vi "CacheConfigFile-SMTPAuthentication.vi"() -> (2 "Authentication Credentials":T1)   [LabVIEW 2020]
uses:
  SMTPCredentials.ctl
  Anemometry Sub Vis/Globals/Constants_global.vi
  <vilib>/Utility/config.llb/Read Key (String).vi
  <vilib>/Utility/config.llb/Write Key (String).vi
  <vilib>/Utility/config.llb/NI_LVConfig.lvlib
panel:
  out "file path":path
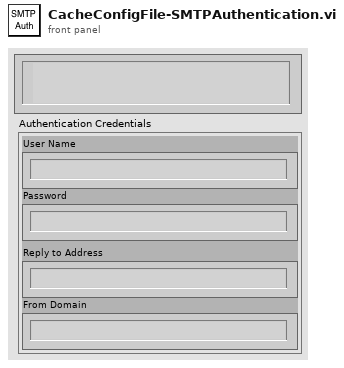
[diagram p1: front panel]
types:
  T1 = typedef "SMTPCredentials.ctl" = cluster{"User Name":string, "Password":string, "Reply to Address":string, "From Domain":string}
  T2 = typedef "NI_LVConfig.lvlib/Config Data RefNum.ctl" = refnum<k1>
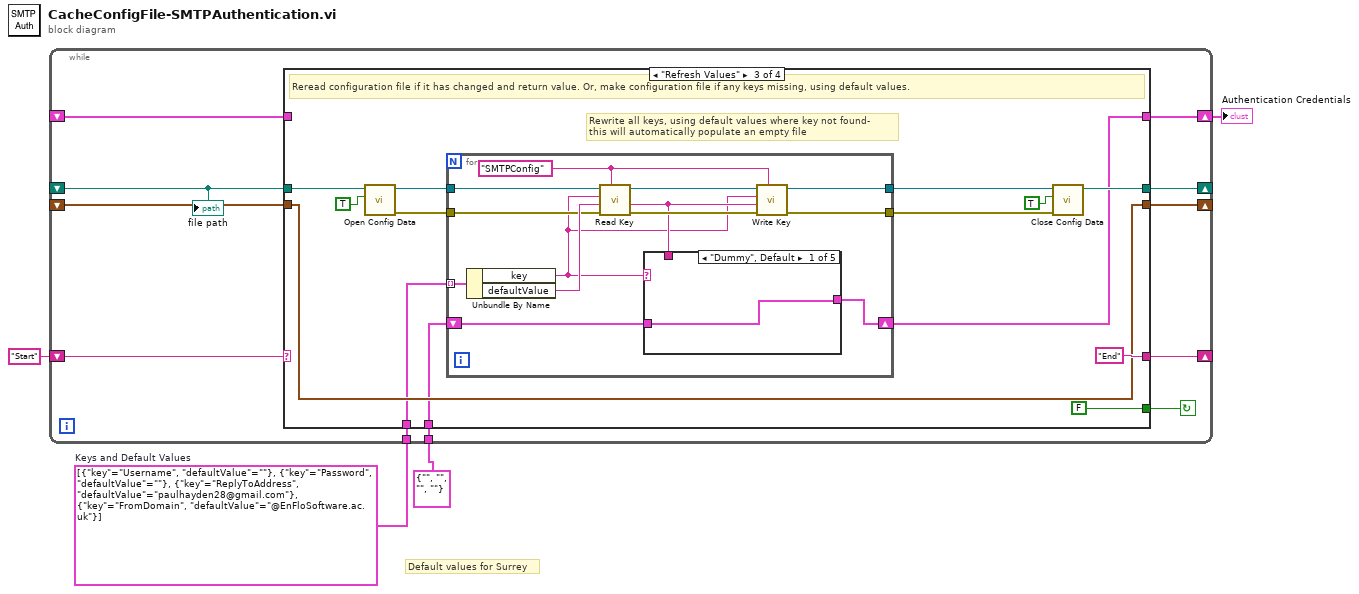
[diagram p0: block diagram]
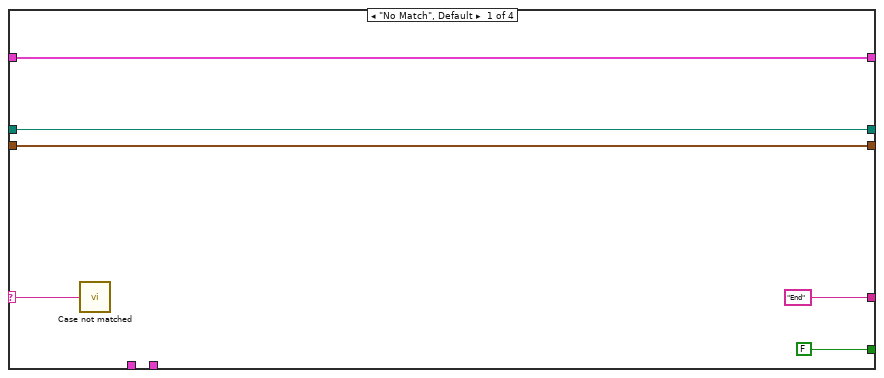
[diagram p2: hidden frame]
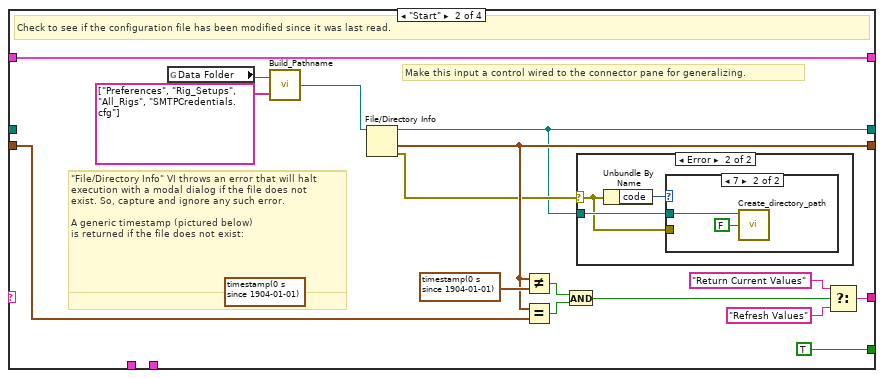
[diagram p3: hidden frame]
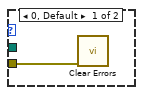
[diagram p5: hidden frame]
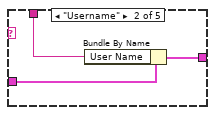
[diagram p6: hidden frame]
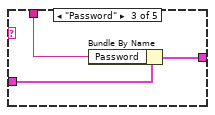
[diagram p7: hidden frame]
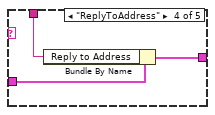
[diagram p8: hidden frame]
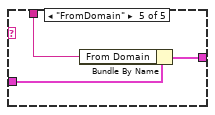
[diagram p9: hidden frame]
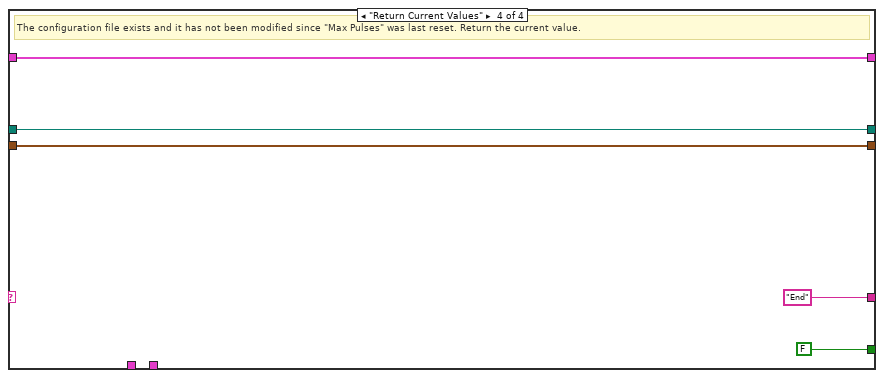
[diagram p10: hidden frame]
diagram:
  w2 = cluster{"key":string, "defaultValue":string}[] [{"key"="Username", "defaultValue"=""}, {"key"="Password", "defaultValue"=""}, {"key"="ReplyToAddress", "defaultValue"="paulhayden28@gmail.com"}, {"key"="FromDomain", "defaultValue"="@EnFloSoftware.ac.uk"}]  # Keys and Default Values
  # "Default values for Surrey"
  n1 = while {
    shift-left: _ -> [w9]
    shift-right: [w11] -> _
    shift-left: _ -> [w10]
    shift-right: [w12] -> w3
    shift-left: "Start" -> [w13]
    shift-right: [w14] -> _
    shift-right: [w8] -> _
    shift-left: _ -> [w7]
    tunnel: w2 -> [w6]
    tunnel: T1 {"User Name"="", "Password"="", "Reply to Address"="", "From Domain"=""} ("Authentication Credentials") -> [w5]
    stop <- w15 continue-if-true
    n2 = case shown="\"Refresh Values\"" w13 {
      selector: w13 -> [w16 _ _ _]
      tunnel: [FALSE TRUE FALSE FALSE] -> w15
      tunnel: ["End" w34 "End" "End"] -> w14
      tunnel: [w19 w37 w44 w88] -> w12
      tunnel: [w18 w31 w51 w87] -> w11
      tunnel: w10 -> [w19 w37 _ w88]
      tunnel: w9 -> [w18 w33 w51 w87]
      tunnel: [w17 w22 w52 w84] -> w8
      tunnel: w7 -> [w17 _ w53 w84]
      tunnel: w6 -> [_ _ w48 _]
      tunnel: w5 -> [_ _ w45 _]
      frame "No Match", Default {
        n3 = call "Case not matched.vi"("Case Name not Matched"=w16) -> ()
      }
      frame "Start" {
        (unwired) "Return Current Values"
        (unwired) timestamp(0 s since 1904-01-01) ("last mod")
        # "Make this input a control wired to the connector pane for generalizing."
        # "Check to see if the configuration file has been modified since it was last read."
        # "\"File/Directory Info\" VI throws an error that will halt execution with a modal dialog if the file does not \nexist. So, make the required directory in this case,\nand ignore other errors until they clearly become\nproblem. (Automatic error handling is disabled for this VI.)\n\nA generic timestamp (pictured below) is returned if the file does not exist:"
        # "\"File/Directory Info\" VI throws an error that will halt execution with a modal dialog if the file does not \nexist. So, capture and ignore any such error.\n\nA generic timestamp (pictured below)\nis returned if the file does not exist:"
        # "\"File/Directory Info\" VI throws an error that will halt execution with a modal dialog if the file does not \nexist. So, capture and ignore any such error.\n\nA generic timestamp (pictured below)\nis returned if the file does not exist:"
        n4 = global read "Constants_global.vi" "Data Folder"() -> (w26:path)
        n5 = call "Build_Pathname.vi"("PathElements"=string[] ["Preferences", "Rig_Setups", "All_Rigs", "SMTPCredentials.cfg"], "PathnameIn"=w26) -> ("AppendedPath"=w25:path)
        n6 = File/Directory Info(path=w25) -> (path out=w22:path, last mod=w31:timestamp, error out=w23:errorcluster)  [unwired: 1 in, 4 out]
        n7 = Not Equal?(x=w31, y=timestamp(0 s since 1904-01-01) ("last mod")) -> (x != y?=w30:bool)
        n8 = Equal?(x=w31, y=w33) -> (x = y?=w29:bool)
        n9 = And(x=w30, y=w29) -> (x .and. y?=w35:bool)
        n10 = case shown="Error" w23 {
          selector: w23 -> [_ w38]
          tunnel: w22 -> [_ w39]
          frame No Error {
          }
          frame Error {
            n11 = Unbundle By Name(w38) -> ("code"=w40:i32)
            n12 = case shown="7" w40 {
              tunnel: w39 -> [_ w42]
              tunnel: w38 -> [w41 _]
              frame 0, Default {
                n13 = call <vilib>:"Clear Errors.vi"("error in (no error)"=w41) -> ()  [unwired: 5 in, 2 out]
              }
              frame 7 {
                n14 = call "Create_directory_path.vi"("Dialog Box"=FALSE, "Path name"=w42) -> ()  [unwired: 1 in, 2 out]
              }
            }
          }
        }
        n15 = Select(t="Return Current Values", s=w35, f="Refresh Values") -> (s? t:f=w34:string)
      }
      frame "Refresh Values" {
        # "Rewrite all keys, using default values where key not found-\nthis will automatically populate an empty file"
        # "Reread configuration file if it has changed and return value. Or, make configuration file if any keys missing, using default values."
        n16 = call <vilib>:"Open Config Data.vi"("create file if necessary (T)"=TRUE, "configuration file path"=w53) -> ("error out"=w47:errorcluster, "refnum"=w55:T2)  [unwired: 7 in, 1 out]
        n17 = for {
          tunnel: w55 -> [w70]
          tunnel: [w68] -> w49
          tunnel: w48 -> [w67] mode=indexing
          tunnel: w47 -> [w65]
          tunnel: [w63] -> w46
          shift-right: [w61] -> w44
          shift-left: w45 -> [w62]
          w59 = "SMTPConfig" ("section")
          n18 = Unbundle By Name(w67) -> ("key"=w58:string, "defaultValue"=w66:string)
          n19 = call-poly <vilib>:"Read Key.vi"("section"=w59, "error in (no error)"=w65, "default value"=w66, "key"=w58, "refnum"=w70) -> ("error out"=w64:errorcluster, "value"=w60:string, "refnum out"=w69:T2)  [unwired: 3 in, 1 out]
          n20 = case shown="\"Dummy\", Default" w58 {
            tunnel: w62 -> [w71 w74 w77 w80 w83]
            tunnel: [w71 w73 w76 w79 w82] -> w61
            tunnel: w60 -> [_ w72 w75 w78 w81]
            frame "Dummy", Default {
            }
            frame "Username" {
              n21 = Bundle By Name(cluster=w74, "User Name"=w72) -> (w73:T1)
            }
            frame "Password" {
              n22 = Bundle By Name(cluster=w77, "Password"=w75) -> (w76:T1)
            }
            frame "ReplyToAddress" {
              n23 = Bundle By Name(cluster=w80, "Reply to Address"=w78) -> (w79:T1)
            }
            frame "FromDomain" {
              n24 = Bundle By Name(cluster=w83, "From Domain"=w81) -> (w82:T1)
            }
          }
          n25 = call-poly <vilib>:"Write Key.vi"("section"=w59, "error in (no error)"=w64, "value"=w60, "key"=w58, "refnum"=w69) -> ("error out"=w63:errorcluster, "refnum out"=w68:T2)  [unwired: 4 in, 1 out]
        }
        n26 = call <vilib>:"Close Config Data.vi"("error in (no error)"=w46, "write file if changed (T)"=TRUE, "refnum"=w49) -> ("file path"=w52:path)  [unwired: 7 in, 1 out]
      }
      frame "Return Current Values" {
        # "The configuration file exists and it has not been modified since \"Max Pulses\" was last reset. Return the current value."
      }
    }
    "file path" <- w7
  }
  "Authentication Credentials" <- w3
